vi "SigMath Class - Append to Window List.vi"(5 "error in (no error)":errorcluster, 7 "GUI VI Ref":refnum<vi>) -> (19 "error out":errorcluster)   [LabVIEW 2020, in "SigMath.lvclass"]
uses:
  SigMath.lvclass
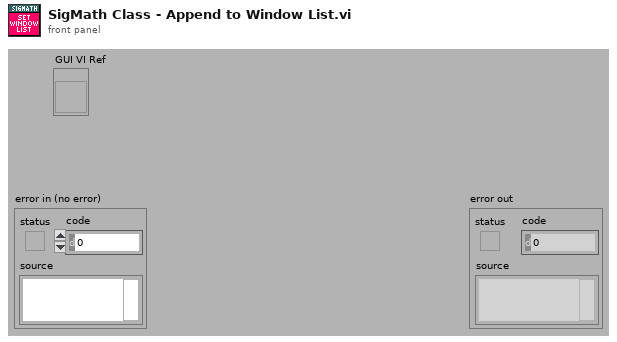
[diagram p1: front panel]
types:
  T1 = typedef "SigMath.lvclass/ClassAttributesRef.ctl" = refnum<data-value>
  T2 = typedef "SigMath.lvclass/ClassAttributes.ctl" = cluster{"Window List":refnum<vi>[]}
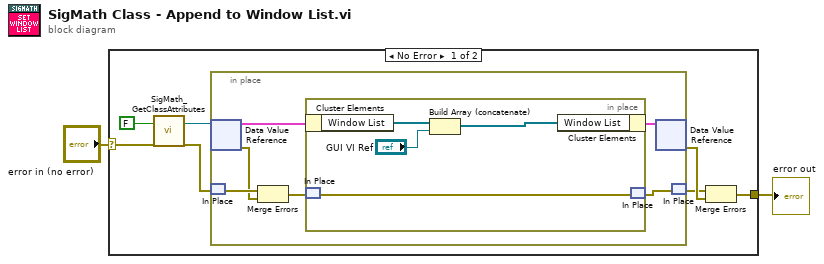
[diagram p0: block diagram]
diagram:
  n1 = case shown="No Error" "error in (no error)" {
    selector: "error in (no error)" -> [w9 w20]
    tunnel: [w7 w20] -> w1
    frame No Error {
      n2 = call "SigMath_GetClassAttributes.vi"("return data? (T)"=FALSE ("return data"), "error in (no error)"=w9) -> ("class attributes ref"=w8:T1, "error out"=w4:errorcluster)  [unwired: 14 in, 2 out]
      n3 = in-place {
        n4 = in-place-dvr #1(w8) -> (w14:T2, w12:errorcluster)
        n5 = in-place-match #2(w4) -> (w13:errorcluster)
        n6 = Merge Errors(w13, w12) -> (w11:errorcluster)
        n7 = in-place {
          n8 = in-place-cluster #3(w14) -> ("Window List"=w19:refnum<vi>[])
          n9 = in-place-match #4(w11) -> (w16:errorcluster)
          n10 = Build Array (concatenate)(w19, "GUI VI Ref") -> (w17:refnum<vi>[])
          n11 = in-place-cluster #3("Window List"=w17) -> (w15:T2)
          n12 = in-place-match #4(w16) -> (w10:errorcluster)
        }
        n13 = in-place-dvr #1(w15) -> (w5:errorcluster)  [unwired: 1 out]
        n14 = in-place-match #2(w10) -> (w3:errorcluster)
      }
      n15 = Merge Errors(w3, w5) -> (w7:errorcluster)
    }
    frame Error {
    }
  }
  "error out" <- w1
